vi "VoltageController.vi"(0 "Y (m)":dbl, 1 "X (m)":dbl, 2 "dBzdt":dbl, 5 "Z (m)":dbl, 7 "dBxdt":dbl, 9 "Bx [T]":dbl, 11 "By [T]":dbl, 12 "Bz [T]":dbl, 13 "dBydt":dbl) -> (3 "XN":dbl, 4 "XP":dbl, 6 "YN":dbl, 10 "YP":dbl, 14 "ZP":dbl, 15 "ZN":dbl)   [LabVIEW 2020]
uses:
  <vilib>/imath/engines/lvmath2/RunTimeEngine/Managers/WorkSpace/UID Generator.vi
  <vilib>/imath/engines/lvmath2/RunTimeEngine/RunTimeType/NIMS_RunTimeType_From StrictType (excl LVString).vi
  <instcachedir>/0/NIMS_RunTimeType_From StrictType (excl LVString)_283B1B2000484AAA8744D21CE97EA49F.lvgen/NIMS_RunTimeType_From StrictType (excl LVString)_283B1B2000484AAA8744D21CE97EA49F_000.vi
  <vilib>/imath/engines/lvmath2/RunTimeEngine/LocalVariableDefStatement/MC_LocalVariableDefStatement_Display.vi
  Documents/LabVIEW Data/MathScriptVIs/MCStatic_53690370032_a09af982989a6940d5e488176ff782fb.vi
  <instcachedir>/0/MCStatic_53690370032_a09af982989a6940d5e488176ff782fb_FB9956AFA4C34A10916D88230AADC989.lvgen/MCStatic_53690370032_a09af982989a6940d5e488176ff782fb_FB9956AFA4C34A10916D88230AADC989_000.vi
  <vilib>/imath/engines/lvmath2/RunTimeEngine/IndexRead/NIMS V(S).vi
  <instcachedir>/0/NIMS V(S)_0488751826AF41519A22953C041130DC.lvgen/NIMS V(S)_0488751826AF41519A22953C041130DC_003.vi
  <vilib>/imath/engines/lvmath2/RunTimeEngine/ErrorHandling/NIMS_Create Error From Enums.vi
  <vilib>/imath/engines/lvmath2/RunTimeEngine/ArithmeticOperatorToken/NIMS_ArithmeticOperator_multmx-internal.vi
  <instcachedir>/0/NIMS_ArithmeticOperator_multmx-internal_B44B9A6937C8407A9A8862E3F2935EB3.lvgen/NIMS_ArithmeticOperator_multmx-internal_B44B9A6937C8407A9A8862E3F2935EB3_003.vi
  <vilib>/imath/engines/lvmath2/RunTimeEngine/ArithmeticOperatorToken/NIMS_ArithmeticOperator_rightdivmx(C,C)-internal.vi
  <instcachedir>/0/NIMS_ArithmeticOperator_rightdivmx(C,C)-internal_4F15F6D1EDF24850BAB8674B5B062781.lvgen/NIMS_ArithmeticOperator_rightdivmx(C,C)-internal_4F15F6D1EDF24850BAB8674B5B062781_000.vi
  <vilib>/imath/engines/lvmath2/RunTimeEngine/ArithmeticOperatorToken/NIMS_ArithmeticOperator_multmx(M,CV)-internal.vi
  <instcachedir>/0/NIMS_ArithmeticOperator_multmx(M,CV)-internal_19A14CC5BE0A4D31BE1E94A2E998D8C3.lvgen/NIMS_ArithmeticOperator_multmx(M,CV)-internal_19A14CC5BE0A4D31BE1E94A2E998D8C3_002.vi
  <instcachedir>/0/NIMS_ArithmeticOperator_multmx(M,CV)-internal_19A14CC5BE0A4D31BE1E94A2E998D8C3.lvgen/NIMS_ArithmeticOperator_multmx(M,CV)-internal_19A14CC5BE0A4D31BE1E94A2E998D8C3_003.vi
  <vilib>/imathl/engines/lvmath/Functions/Error Handling/Create Error.vi
  <vilib>/imath/engines/lvmath2/RunTimeEngine/Managers/SymbolTable/Clear UID.vi
  <vilib>/imath/engines/lvmath2/RunTimeEngine/NodeEndStatement/NIMS_NodeEndStatement_Output.vi
  <instcachedir>/0/NIMS_NodeEndStatement_Output_53EC0D466D134D7ABD903AC30B43404B.lvgen/NIMS_NodeEndStatement_Output_53EC0D466D134D7ABD903AC30B43404B_009.vi
  <vilib>/imath/engines/lvmath2/RunTimeEngine/ErrorHandling/NIMS_Finalize Error.vi
  MatlabFunctions/GFunction.m
  <vilib>/imath/engines/lvmath2/RunTimeEngine/Managers/SymbolTable/NIMS_WorkSpace.lvlib
panel:
  # "Current in each coil (A)"
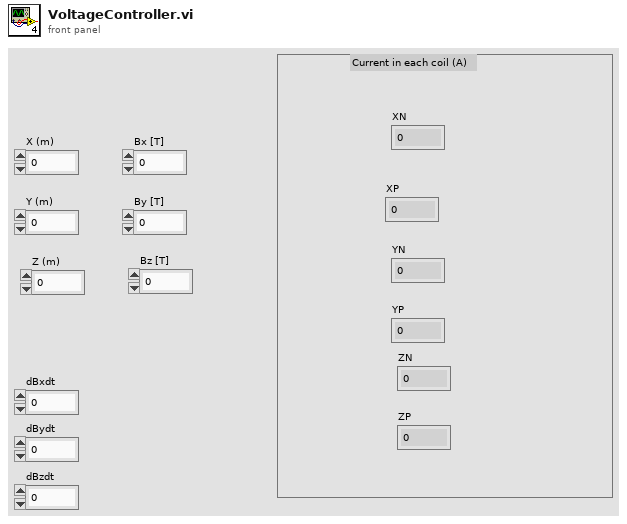
[diagram p1: front panel]
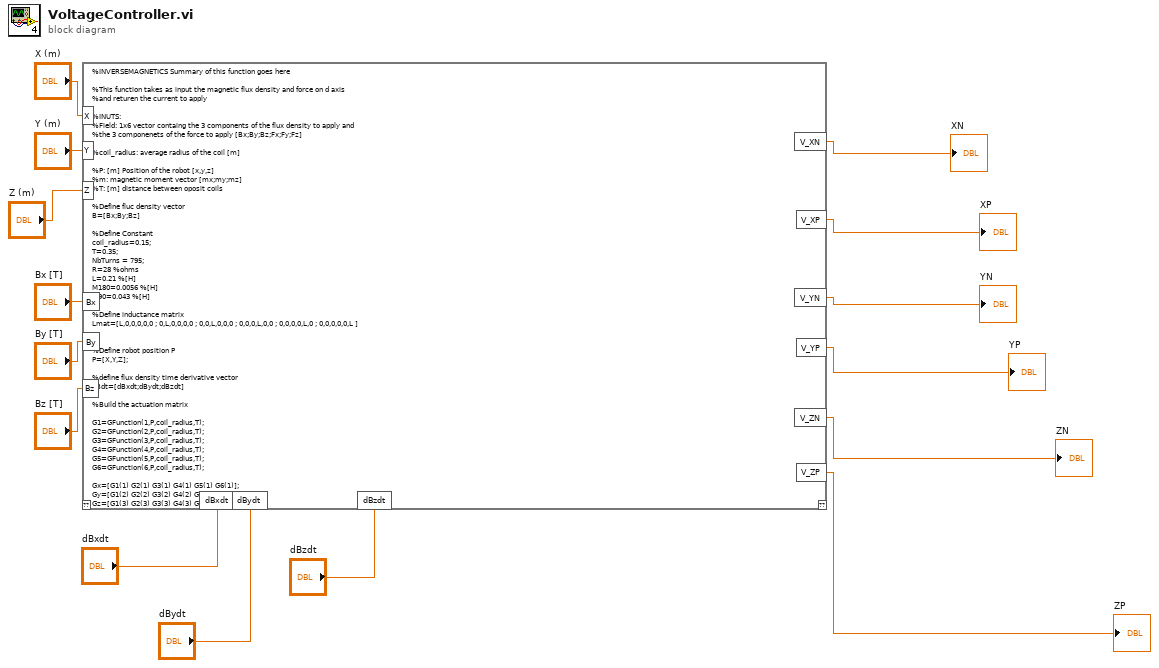
[diagram p0: block diagram]
diagram:
  n1 = mathscript code="%INVERSEMAGNETICS Summary of this function goes here\n\n%This function takes as input the magnetic flux density and force on d axis\n%and returen the current to apply\n\n%INUTS: \n%Field: 1x6 vector containg the 3 components of the flux density to apply and\n%the 3 componenets of the force to apply [Bx;By;Bz;Fx;Fy;Fz]\n\n%coil_radius: average radius of the coil [m]\n\n%P: [m] Position of the robot [x,y,z]\n%m: magnetic moment vector [mx;my;mz]\n%T: [m] distance between oposit coils\n\n%Define fluc density vector\nB=[Bx;By;Bz]\n\n%Define Constant\ncoil_radius=0.15;\nT=0.35;\nNbTurns = 795;\nR=28 %ohms\nL=0.21 %[H]\nM180=0.0056 %[H]\nM90=0.043 %[H]\n\n%Define inductance matrix\nLmat=[L,0,0,0,0,0 ; 0,L,0,0,0,0 ; 0,0,L,0,0,0 ; 0,0,0,L,0,0 ; 0,0,0,0,L,0 ; 0,0,0,0,0,L ]\n\n\n%Define robot position P\nP=[X,Y,Z];\n\n%define flux density time derivative vector\ndBdt=[dBxdt;dBydt;dBzdt]\n\n%Build the actuation matrix \n\nG1=GFunction(1,P,coil_radius,T);\nG2=GFunction(2,P,coil_radius,T);\nG3=GFunction(3,P,coil_radius,T);\nG4=GFunction(4,P,coil_radius,T);\nG5=GFunction(5,P,coil_radius,T);\nG6=GFunction(6,P,coil_radius,T);\n\nGx=[G1(1) G2(1) G3(1) G4(1) G5(1) G6(1)];\nGy=[G1(2) G2(2) G3(2) G4(2) G5(2) G6(2)];\nGz=[G1(3) G2(3) G3(3) G4(3) G5(3) G6(3)];\n\n%Actuation Matrix\nA=[Gx;Gy;Gz];\n\n%Inverse the matrix and return the current\n\n\nI=A'/(A*A')*[Bx;By;Bz]./NbTurns;\ndIdt=A'/(A*A')*dBdt./NbTurns;\nV=R*I+Lmat*dIdt\n\nV_XP =V(2);\nV_XN =V(1);\nV_YP =V(4);\nV_YN =V(3);\nV_ZP =-V(6);\nV_ZN =-V(5);"("X"="X (m)", "Y"="Y (m)", "Z"="Z (m)", "Bx"="Bx [T]", "By"="By [T]", "Bz"="Bz [T]", "dBxdt"="dBxdt", "dBydt"="dBydt", "dBzdt"="dBzdt") -> ("V_XP"=→"XP":cdb, "V_YN"=→"YN":cdb, "V_YP"=→"YP":cdb, "V_ZP"=→"ZP":cdb, "V_ZN"=→"ZN":cdb, "V_XN"=→"XN":cdb)  [unwired: 1 in, 1 out]
